vi "Link.vi"(0 "Termination in":refnum<class "Termination.lvclass">, 7 "State names":string[](array[string]), 9 "Event names":string[](array[string]), 11 "error in (no error)":errorcluster) -> (4 "Termination out":refnum<class "Termination.lvclass">, 15 "error out":errorcluster)   [LabVIEW 2020, in "Termination.lvclass"]
uses:
  Termination.lvclass
  Termination.lvclass/Termination.ctl
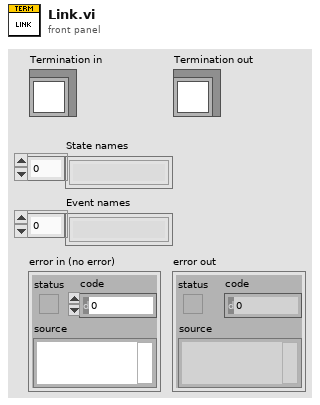
[diagram p1: front panel]
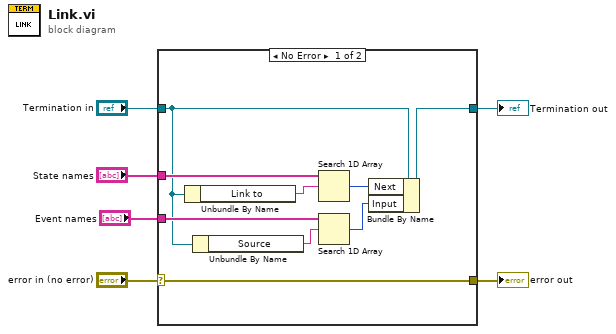
[diagram p0: block diagram]
diagram:
  n1 = case shown="No Error" "error in (no error)" {
    selector: "error in (no error)" -> [w15 w17]
    tunnel: [w15 w17] -> w5
    tunnel: [w14 w16] -> w3
    tunnel: "Termination in" -> [w9 w16]
    tunnel: "State names" -> [w13 _]
    tunnel: "Event names" -> [w10 _]
    frame No Error {
      n2 = Unbundle By Name(w9) -> ("Link to"=w12:string)
      n3 = Unbundle By Name(w9) -> ("Source"=w8:string)
      n4 = Search 1D Array(1D array=w13, element=w12) -> (index of element=w11:i32)  [unwired: 1 in]
      n5 = Search 1D Array(1D array=w10, element=w8) -> (index of element=w7:i32)  [unwired: 1 in]
      n6 = Bundle By Name(cluster=w9, "Next"=w11, "Input"=w7) -> (w14:refnum<class "Termination.lvclass">)
    }
    frame Error {
    }
  }
  "error out" <- w5
  "Termination out" <- w3
